vi "HP3458A Close.vi"(8 "error in (no error)":errorcluster, 11 "VISA in":refnum<visa-resource-name>) -> (0 "error out":errorcluster)   [LabVIEW 2020]
uses:
  <vilib>/Instr/_visa.llb/VISA GPIB Control REN Mode.ctl
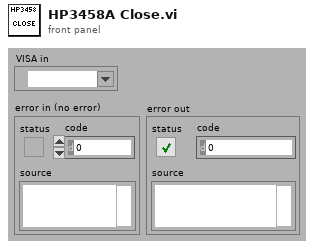
[diagram p1: front panel]
types:
  T1 = typedef "VISA GPIB Control REN Mode.ctl" = u16
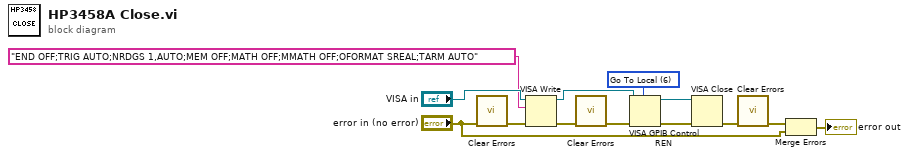
[diagram p0: block diagram]
diagram:
  w7 = T1 6 items=["Deassert REN", "Assert REN", "Go To Local; Deassert REN ", "Assert REN; Address Device", "Local Lockout (Addressed Devices)", "Local Lockout (This Device)", "Go To Local"] ("Mode")
  n1 = call <vilib>:"Clear Errors.vi"("error in (no error)"="error in (no error)") -> ("error out"=w4:errorcluster)  [unwired: 5 in, 1 out]
  n2 = VISA Write(VISA resource name="VISA in", write buffer="END OFF;TRIG AUTO;NRDGS 1,AUTO;MEM OFF;MATH OFF;MMATH OFF;OFORMAT SREAL;TARM AUTO", error in (no error)=w4) -> (VISA resource name out=w2:refnum<visa-resource-name>, error out=w5:errorcluster)  [unwired: 1 out]
  n3 = call <vilib>:"Clear Errors.vi"("error in (no error)"=w5) -> ("error out"=w6:errorcluster)  [unwired: 5 in, 1 out]
  n4 = VISA GPIB Control REN(8:w6, 10:w7, 11:w2) -> (0:w9:errorcluster, 3:w8:refnum<visa-resource-name>)
  n5 = VISA Close(VISA resource name=w8, error in (no error)=w9) -> (error out=w13:errorcluster)
  n6 = call <vilib>:"Clear Errors.vi"("error in (no error)"=w13) -> ("error out"=w12:errorcluster)  [unwired: 5 in, 1 out]
  n7 = Merge Errors(w12, "error in (no error)") -> (→"error out":errorcluster)
